vi "Read condtional.vi"(9 "LoopTunnel in":refnum<class "LoopTunnel.lvclass">) -> (3 "LoopTunnel out":refnum<class "LoopTunnel.lvclass">, 4 "condtional":bool)   [LabVIEW 2014, in "LoopTunnel.lvclass"]
uses:
  LoopTunnel.lvclass
  LoopTunnel.lvclass/LoopTunnel.ctl
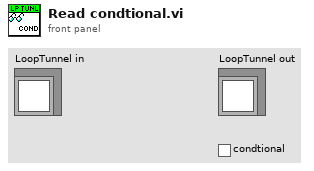
[diagram p1: front panel]
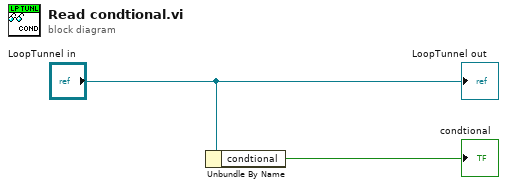
[diagram p0: block diagram]
diagram:
  n1 = Unbundle By Name("LoopTunnel in") -> ("condtional"=→"condtional":bool)
  "LoopTunnel out" <- "LoopTunnel in"
